vi "Matrix To Array - RM.vi"(1 "Real Matrix":T1) -> (0 "Real 2D Array":dbl[][](array[numeric]))   [LabVIEW 2020, in "NI_Matrix.lvlib"]
doc: "Converts a matrix of elements to an array of elements of the same data type. Wire data to the <B>Real Matrix</B> input to determine the polymorphic instance to use or manually select the instance."
uses:
  NI_Matrix.lvlib
  RealMatrix.ctl
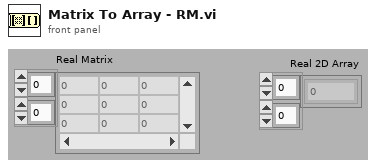
[diagram p1: front panel]
types:
  T1 = typedef "NI_Matrix.lvlib/RealMatrix.ctl" = dbl[][]
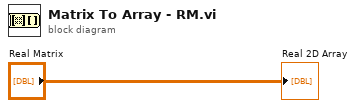
[diagram p0: block diagram]
diagram:
  "Real 2D Array" <- "Real Matrix"
